vi "Wyznaczenie azymutu na podstawie współrzędnych geograficznych.vi"(7 "Azymut robota\n pocz/nowy":dbl caption="Azymut robota pocz/nowy" min=0.0 max=360.0, 9 "latitude":dbl, 10 "Longitude":dbl) -> (3 "Azymut robota\n pocz/nowy 2":dbl)   [LabVIEW 2015, in "Biblioteka moduł map v3.lvlib" / "Pomocnicze.lvlib"]
doc: "Zadaniem pliku jest wyznaczenie odległości robota od punktu startowego na podstawie znanych współrzędnych geograficznych pliku startowego oraz odczytów z odbiornika GPS."
uses:
  Pomocnicze.lvlib
  Matematyczne/Matematyczne.lvlib
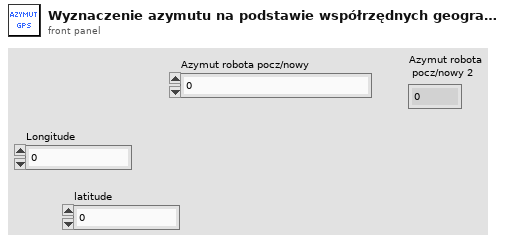
[diagram p1: front panel]
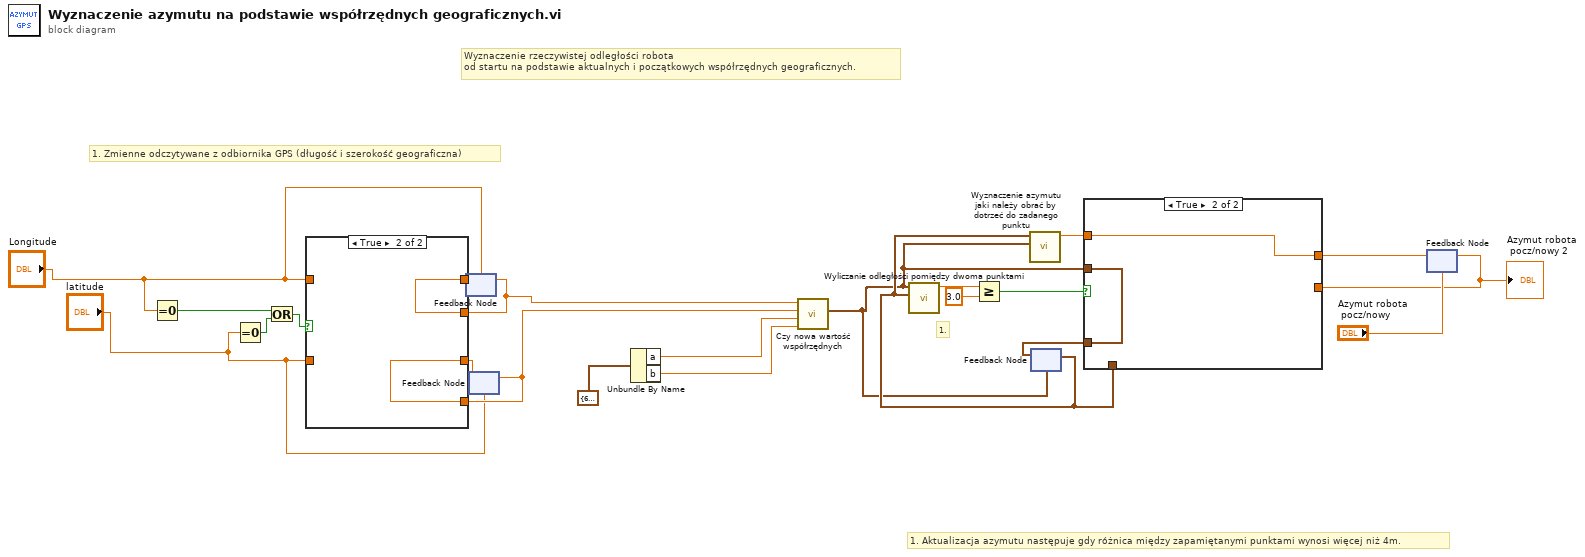
[diagram p0: block diagram]
diagram:
  # "1. Aktualizacja azymutu następuje gdy różnica między zapamiętanymi punktami wynosi więcej niż 4m."
  # "1."
  # "Wyznaczenie rzeczywistej odległości robota \nod startu na podstawie aktualnych i początkowych współrzędnych geograficznych."
  # "1. Zmienne odczytywane z odbiornika GPS (długość i szerokość geograficzna)"
  n1 = Equal To 0?(x="Longitude") -> (x = 0?=w10:bool)
  n2 = Equal To 0?(x="latitude") -> (x = 0?=w9:bool)
  n3 = Or(x=w10, y=w9) -> (x .or. y?=w8:bool)
  n4 = feedback #1("Longitude") -> (w5:dbl)
  n5 = feedback #2("latitude") -> (w4:dbl)
  n6 = case shown="True" w8 {
    tunnel: [w24 w26] -> w7
    tunnel: "Longitude" -> [w24 _]
    tunnel: "latitude" -> [w23 _]
    tunnel: [w23 w25] -> w6
    tunnel: w5 -> [_ w26]
    tunnel: w4 -> [_ w25]
    frame False {
    }
    frame True {
    }
  }
  n7 = feedback-in #1(w7) -> ()
  n8 = feedback-in #2(w6) -> ()
  n9 = Unbundle By Name(cluster{"a":dbl, "b":dbl} {"a"=6378137.0, "b"=6356752.3142} ("Parametry odwzorowania Ziemi (WGS84)")) -> ("a"=w20:dbl, "b"=w21:dbl)
  n10 = call "Czy nowa wartość współrzędnych.vi"("b"=w21, "a"=w20, "szerokość geograficzna"=w4, "Długość geograficzna"=w5) -> ("Położenie"=w12:cluster{"X/E [m]":dbl, "Y/N [m]":dbl})  [unwired: 5 in, 2 out]
  n11 = feedback #3(w12) -> (w13:cluster{"X/E [m]":dbl, "Y/N [m]":dbl})
  n12 = call "Wyliczanie odległości pomiędzy dwoma punktami.vi"("Polozenie 1"=w13, "Polozenie in"=w12) -> ("Numeric"=w19:dbl)  [unwired: 9 in]
  n13 = Greater Or Equal?(x=w19, y=3.0) -> (x >= y?=w17:bool)
  n14 = call "Wyznaczenie azymutu jaki należy obrać by dotrzeć do zadanego punktu.vi"("Położenie końcowe"=w12, "Położenie aktualne"=w13) -> ("Azymut"=w16:dbl)  [unwired: 9 in]
  n15 = feedback #4("Azymut robota\n pocz/nowy") -> (w3:dbl)
  "Azymut robota\n pocz/nowy 2" <- w3
  n16 = case shown="True" w17 {
    tunnel: [w27 w30] -> w15
    tunnel: w16 -> [_ w30]
    tunnel: [w28 w29] -> w14
    tunnel: w12 -> [_ w29]
    tunnel: w13 -> [w28 _]
    tunnel: w3 -> [w27 _]
    frame False {
    }
    frame True {
    }
  }
  n17 = feedback-in #3(w14) -> ()
  n18 = feedback-in #4(w15) -> ()
